vi "Initialize.vi"(8 "error in":errorcluster, 9 "Number of Channels":u32=1, 10 "Plugin Name":string, 11 "Current Control in":refnum<class "Current Control.lvclass">) -> (0 "error out":errorcluster, 3 "Current Control out":refnum<class "Current Control.lvclass">)   [LabVIEW 2023, in "Current Control.lvclass"]
uses:
  Current Control.lvclass
  Current Control.lvclass/Current Control.ctl
  <vilib>/ADAS Replay HIL/Channels/Tag Wrapper/Polymorphic/Open Consumer Tag (Double).vi
  <vilib>/ADAS Replay HIL/Channels/Tag Wrapper/Polymorphic/Open Consumer Tag (Double).vi/bacb721e-673a-491a-accd-959f2e1f334e.vi
  <vilib>/ADAS Replay HIL/Channels/Tag Wrapper/Polymorphic/Open Consumer Tag (Double).vi/bacb721e-673a-491a-accd-959f2e1f334e.vi/c28b0ead-42ad-4072-80a2-aca7f2bd7ce3.vi
  <vilib>/ADAS Replay HIL/AdasHilServices/AdasHilServices Fill In Error Info Ex.vi
  <vilib>/ADAS Replay HIL/Channels/Tag Wrapper/Tag Wrapper.lvlib
  Utilities/Utilities.lvlib
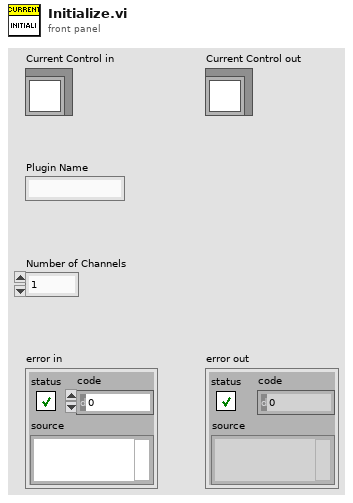
[diagram p1: front panel]
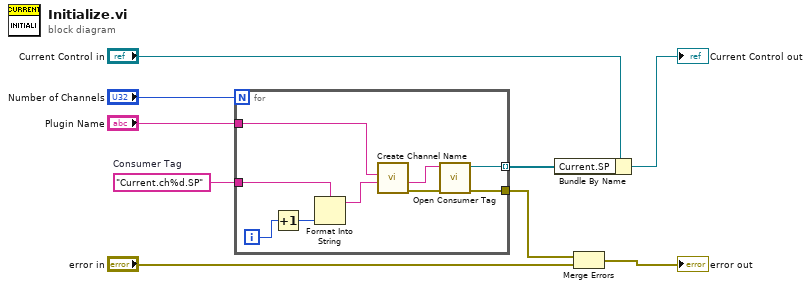
[diagram p0: block diagram]
diagram:
  w3 = "Current.ch%d.SP"  # Consumer Tag
  n1 = for {
    N: "Number of Channels" -> [_]
    tunnel: [w18] -> w9 mode=indexing
    tunnel: [w17] -> w5
    tunnel: w3 -> [w12]
    tunnel: "Plugin Name" -> [w15]
    i -> [w11]
    n2 = Increment(x=w11) -> (x+1=w10:i32)
    n3 = Format Into String(format string=w12, w10) -> (resulting string=w13:string)  [unwired: 2 in, 1 out]
    n4 = call "Create Channel Name.vi"("Channel Name"=w13, "Plugin Name"=w15) -> ("error out"=w14:errorcluster, "Data Channel Name"=w16:string)  [unwired: 8 in]
    n5 = call-poly <vilib>:"Open Consumer Tag.vi"("error in"=w14, "Channel Name"=w16) -> ("error out"=w17:errorcluster, "ADAS HIL Channel"=w18:refnum<k21>)  [unwired: 8 in]
  }
  n6 = Bundle By Name(cluster="Current Control in", "Current.SP"=w9) -> (→"Current Control out":refnum<class "Current Control.lvclass">)
  n7 = Merge Errors(w5, "error in") -> (→"error out":errorcluster)
